vi "Set Valve Mode.vi"(8 "error in (no error)":errorcluster, 10 "valve mode":u8(ring) items=["auto", "open", "closed"], 11 "RRG in":refnum<class "Eltochpribor RRG.lvclass">) -> (0 "error out":errorcluster, 3 "RRG out":refnum<class "Eltochpribor RRG.lvclass">)   [LabVIEW 2015, in "Eltochpribor RRG.lvclass"]
doc: "Sets valve mode (automatic flow regulation/open/closed)."
uses:
  Eltochpribor RRG.lvclass
  Modbus Client/PL Modbus Client.lvclass
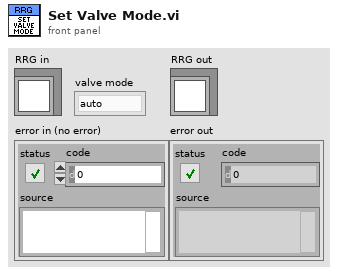
[diagram p1: front panel]
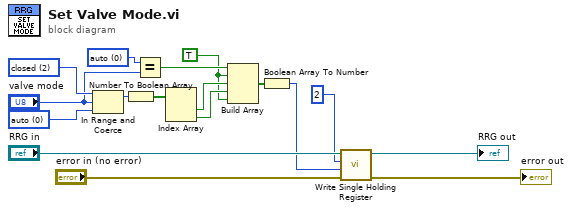
[diagram p0: block diagram]
diagram:
  w3 = TRUE ("element")
  w8 = u8 0 items=["auto", "open", "closed"] ("valve mode")
  w12 = u8 2 items=["auto", "open", "closed"] ("valve mode")
  w11 = u8 0 items=["auto", "open", "closed"] ("valve mode")
  n1 = In Range and Coerce(upper limit=w12, x="valve mode", lower limit=w11) -> (coerced(x)=w10:u8)  [unwired: 1 out]
  n2 = Number To Boolean Array(number=w10) -> (Boolean array=w6:bool[])
  n3 = Equal?(x=w8, y="valve mode") -> (x = y?=w7:bool)
  n4 = Index Array(array=w6) -> (element #1=w5:bool, element #2=w4:bool)  [unwired: 2 in]
  n5 = Build Array(w7, w3, w5, w4, w3) -> (w2:bool[])
  n6 = Boolean Array To Number(Boolean array=w2) -> (number=w1:u32)
  n7 = call "Write Single Holding Register.vi"("error in (no error)"="error in (no error)", "value"=w1, "address"=u16 2, "MODBUS in"="RRG in") -> ("error out"=→"error out":errorcluster, "MODBUS out"=→"RRG out":refnum<class "Eltochpribor RRG.lvclass">)  [unwired: 6 in]
